vi "Agilent VNA Set Measurement.vi"(4 "Trace":i8=1 min=1 max=99 step=1, 5 "Parameter":T1 {"Stimulus Port" min=1 step=1; "Response Port" min=1 step=1}, 6 "Channel":i8=1 min=1 max=99 step=1, 7 "Agilent VNA":T2, 8 "error in (no error)":errorcluster, 9 "Conversion (Off)":T3, 10 "Measurement (SXX)":T4=enum."Analog In - Aux In", 11 "VISA Resource Name":refnum<visa-resource-name>) -> (0 "error out":errorcluster, 3 "dup VISA Resource Name":refnum<visa-resource-name>)   [LabVIEW 2011]
doc: "This VI for the HP8753B Network Analyzer sets the measurement."
uses:
  TypeDefs/Agilent VNA Measurement.ctl
  TypeDefs/Agilent VNA Conversion.ctl
  TypeDefs/Agilent VNA Instrument Info.ctl
  tests/S Parameter/TypeDefs/SP Parameter.ctl
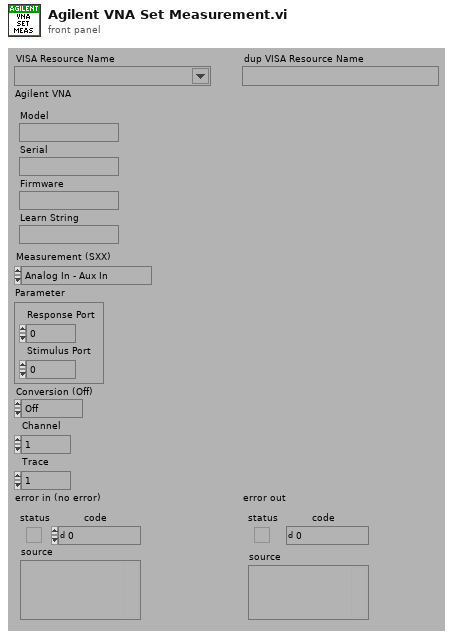
[diagram p1: front panel]
types:
  T1 = typedef "SP Parameter.ctl" = cluster{"Stimulus Port":i8, "Response Port":i8}
  T2 = typedef "Agilent VNA Instrument Info.ctl" = cluster{"Model":string, "Serial":string, "Firmware":string, "Learn String":string}
  T3 = typedef "Agilent VNA Conversion.ctl" = enum16{"Off", "Z Reflection", "Z Transmit", "Y Reflection", "Y Transmit", "Inversion", "ZT Shunt", "YT Shunt", "Conjugation"}
  T4 = typedef "Agilent VNA Measurement.ctl" = enum32{"SXX", "Analog In - Aux In", "A/R", "B/R", "A/B", "A", "B", "R"}
  T5 = typedef "Agilent VNA Model.ctl" = enum16{"Not Supported", "8510X", "8719X", "8720X", "8722X", "8753X", "ENA", "PNA", "Field Fox"}
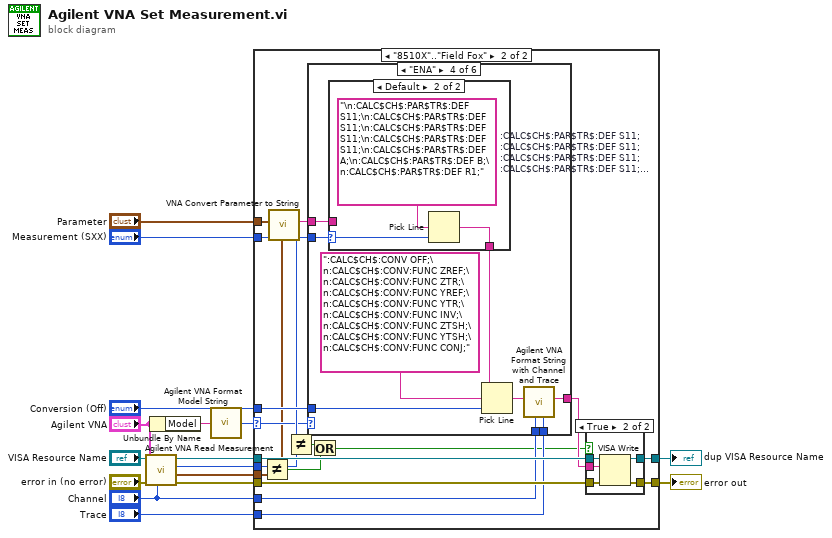
[diagram p0: block diagram]
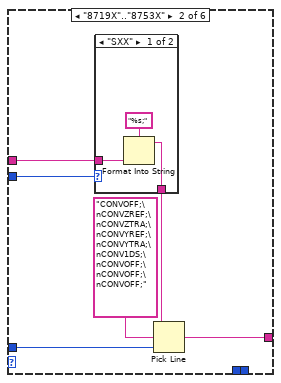
[diagram p4: hidden frame]
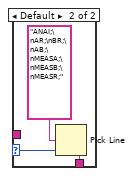
[diagram p5: hidden frame]
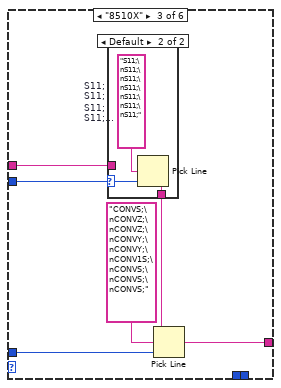
[diagram p6: hidden frame]
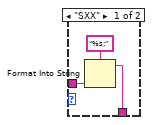
[diagram p7: hidden frame]
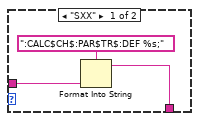
[diagram p8: hidden frame]
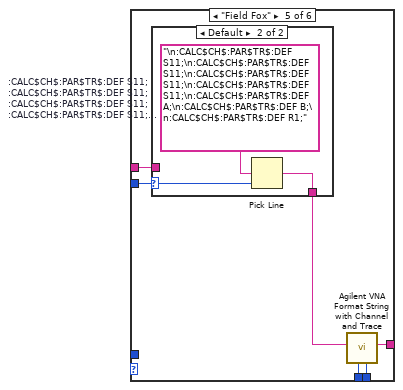
[diagram p9: hidden frame]
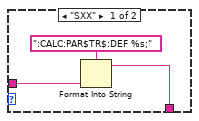
[diagram p10: hidden frame]
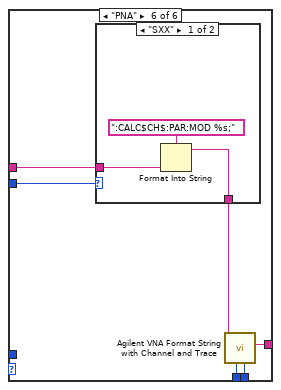
[diagram p11: hidden frame]
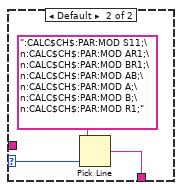
[diagram p12: hidden frame]
diagram:
  n1 = call "Agilent VNA Read Measurement.vi"("Channel"="Channel", "Agilent VNA"="Agilent VNA", "error in (no error)"="error in (no error)", "VISA Resource Name"="VISA Resource Name") -> ("error out"=w12:errorcluster, "Parameter"=w1:T1, "Measurement"=w11:T4, "dup VISA Resource Name"=w13:refnum<visa-resource-name>)  [unwired: 4 out]
  n2 = Unbundle By Name("Agilent VNA") -> ("Model"=w6:string)
  n3 = call "Agilent VNA Format Model String.vi"("Model"=w6) -> ("Model"=w2:T5)
  n4 = case shown="\"8510X\"..\"Field Fox\"" w2 {
    selector: w2 -> [_ w24]
    tunnel: "Conversion (Off)" -> [_ w35]
    tunnel: w13 -> [w18 w34]
    tunnel: w12 -> [w17 w33]
    tunnel: w11 -> [_ w32]
    tunnel: "Channel" -> [_ w31]
    tunnel: "Trace" -> [_ w30]
    tunnel: "Measurement (SXX)" -> [_ w29]
    tunnel: "Parameter" -> [_ w23]
    tunnel: [w18 w26] -> w4
    tunnel: [w17 w25] -> w3
    tunnel: w1 -> [_ w22]
    frame "Not Supported" {
    }
    frame "8510X".."Field Fox" {
      n5 = Not Equal?(x=w23, y=w22) -> (x != y?=w21:bool)
      n6 = call "VNA Convert Parameter to String.vi"("Parameter"=w23) -> ("Parameter String"=w27:string)  [unwired: 10 out]
      n7 = Not Equal?(x=w29, y=w32) -> (x != y?=w20:bool)
      n8 = case shown="\"ENA\"" w24 {
        tunnel: w35 -> [_ w41 w53 w68 _ _]
        tunnel: [_ w39 w51 w65 w80 w92] -> w28
        tunnel: w29 -> [_ w37 w49 w61 w77 w88]
        tunnel: w30 -> [_ _ _ w63 w79 w91]
        tunnel: w31 -> [_ _ _ w62 w78 w89]
        tunnel: w27 -> [_ w36 w48 w60 w76 w87]
        frame "Not Supported" {
        }
        frame "8719X".."8753X" {
          n9 = case shown="\"SXX\"" w37 {
            selector: w37 -> [_ w45]
            tunnel: [w42 w46] -> w38
            tunnel: w36 -> [w43 _]
            frame "SXX" {
              n10 = Format Into String(format string="%s;", w43) -> (resulting string=w42:string)  [unwired: 2 in, 1 out]
            }
            frame Default {
              n11 = Pick Line(multi-line string="ANAI;\nAR;\nBR;\nAB;\nMEASA;\nMEASB;\nMEASR;", line index=w45) -> (output string=w46:string)  [unwired: 1 out]
            }
          }
          n12 = Pick Line(string ("")=w38, multi-line string="CONVOFF;\nCONVZREF;\nCONVZTRA;\nCONVYREF;\nCONVYTRA;\nCONV1DS;\nCONVOFF;\nCONVOFF;\nCONVOFF;", line index=w41) -> (output string=w39:string)
        }
        frame "8510X" {
          n13 = case shown="Default" w49 {
            selector: w49 -> [_ w57]
            tunnel: [w55 w58] -> w50
            tunnel: w48 -> [w54 _]
            frame "SXX" {
              n14 = Format Into String(format string="%s;", w54) -> (resulting string=w55:string)  [unwired: 2 in, 1 out]
            }
            frame Default {
              w59 = "S11;\nS11;\nS11;\nS11;\nS11;\nS11;\nS11;"  # S11; S11; S11; S11; S11; S11; S11;
              n15 = Pick Line(multi-line string=w59, line index=w57) -> (output string=w58:string)  [unwired: 1 out]
            }
          }
          n16 = Pick Line(string ("")=w50, multi-line string="CONVS;\nCONVZ;\nCONVZ;\nCONVY;\nCONVY;\nCONV1S;\nCONVS;\nCONVS;\nCONVS;", line index=w53) -> (output string=w51:string)
        }
        frame "ENA" {
          n17 = case shown="Default" w61 {
            selector: w61 -> [_ w72]
            tunnel: [w70 w73] -> w64
            tunnel: w60 -> [w69 _]
            frame "SXX" {
              n18 = Format Into String(format string=":CALC$CH$:PAR$TR$:DEF %s;", w69) -> (resulting string=w70:string)  [unwired: 2 in, 1 out]
            }
            frame Default {
              w74 = "\n:CALC$CH$:PAR$TR$:DEF S11;\n:CALC$CH$:PAR$TR$:DEF S11;\n:CALC$CH$:PAR$TR$:DEF S11;\n:CALC$CH$:PAR$TR$:DEF S11;\n:CALC$CH$:PAR$TR$:DEF A;\n:CALC$CH$:PAR$TR$:DEF B;\n:CALC$CH$:PAR$TR$:DEF R1;"  # :CALC$CH$:PAR$TR$:DEF S11; :CALC$CH$:PAR$TR$:DEF S11; :CALC$CH$:PAR$TR$:DEF S11; :CALC$CH$:PAR$TR$:DEF S11; :CALC$CH$:PAR$TR$:DEF A; :CALC$CH$:PAR$TR$:DEF B; :CALC$CH$:PAR$TR$:DEF R1;
              n19 = Pick Line(multi-line string=w74, line index=w72) -> (output string=w73:string)  [unwired: 1 out]
            }
          }
          n20 = Pick Line(string ("")=w64, multi-line string=":CALC$CH$:CONV OFF;\n:CALC$CH$:CONV:FUNC ZREF;\n:CALC$CH$:CONV:FUNC ZTR;\n:CALC$CH$:CONV:FUNC YREF;\n:CALC$CH$:CONV:FUNC YTR;\n:CALC$CH$:CONV:FUNC INV;\n:CALC$CH$:CONV:FUNC ZTSH;\n:CALC$CH$:CONV:FUNC YTSH;\n:CALC$CH$:CONV:FUNC CONJ;", line index=w68) -> (output string=w66:string)
          n21 = call "Agilent VNA Format String with Channel and Trace.vi"("Trace"=w63, "Channel"=w62, "String"=w66) -> ("String Out"=w65:string)  [unwired: 6 out]
        }
        frame "Field Fox" {
          n22 = case shown="Default" w77 {
            selector: w77 -> [_ w84]
            tunnel: [w82 w85] -> w75
            tunnel: w76 -> [w81 _]
            frame "SXX" {
              n23 = Format Into String(format string=":CALC:PAR$TR$:DEF %s;", w81) -> (resulting string=w82:string)  [unwired: 2 in, 1 out]
            }
            frame Default {
              w86 = "\n:CALC$CH$:PAR$TR$:DEF S11;\n:CALC$CH$:PAR$TR$:DEF S11;\n:CALC$CH$:PAR$TR$:DEF S11;\n:CALC$CH$:PAR$TR$:DEF S11;\n:CALC$CH$:PAR$TR$:DEF A;\n:CALC$CH$:PAR$TR$:DEF B;\n:CALC$CH$:PAR$TR$:DEF R1;"  # :CALC$CH$:PAR$TR$:DEF S11; :CALC$CH$:PAR$TR$:DEF S11; :CALC$CH$:PAR$TR$:DEF S11; :CALC$CH$:PAR$TR$:DEF S11; :CALC$CH$:PAR$TR$:DEF A; :CALC$CH$:PAR$TR$:DEF B; :CALC$CH$:PAR$TR$:DEF R1;
              n24 = Pick Line(multi-line string=w86, line index=w84) -> (output string=w85:string)  [unwired: 1 out]
            }
          }
          n25 = call "Agilent VNA Format String with Channel and Trace.vi"("Trace"=w79, "Channel"=w78, "String"=w75) -> ("String Out"=w80:string)  [unwired: 6 out]
        }
        frame "PNA" {
          n26 = case shown="\"SXX\"" w88 {
            selector: w88 -> [_ w96]
            tunnel: [w93 w97] -> w90
            tunnel: w87 -> [w94 _]
            frame "SXX" {
              n27 = Format Into String(format string=":CALC$CH$:PAR:MOD %s;", w94) -> (resulting string=w93:string)  [unwired: 2 in, 1 out]
            }
            frame Default {
              n28 = Pick Line(multi-line string=":CALC$CH$:PAR:MOD S11;\n:CALC$CH$:PAR:MOD AR1;\n:CALC$CH$:PAR:MOD BR1;\n:CALC$CH$:PAR:MOD AB;\n:CALC$CH$:PAR:MOD A;\n:CALC$CH$:PAR:MOD B;\n:CALC$CH$:PAR:MOD R1;", line index=w96) -> (output string=w97:string)  [unwired: 1 out]
            }
          }
          n29 = call "Agilent VNA Format String with Channel and Trace.vi"("Trace"=w91, "Channel"=w89, "String"=w90) -> ("String Out"=w92:string)  [unwired: 6 out]
        }
      }
      n30 = Or(x=w20, y=w21) -> (x .or. y?=w19:bool)
      n31 = case shown="True" w19 {
        tunnel: w28 -> [_ w105]
        tunnel: [w99 w104] -> w26
        tunnel: [w100 w103] -> w25
        tunnel: w34 -> [w99 w102]
        tunnel: w33 -> [w100 w101]
        frame False {
        }
        frame True {
          n32 = VISA Write(VISA resource name=w102, write buffer=w105, error in (no error)=w101) -> (VISA resource name out=w104:refnum<visa-resource-name>, error out=w103:errorcluster)  [unwired: 1 out]
        }
      }
    }
  }
  "dup VISA Resource Name" <- w4
  "error out" <- w3
